vi "TREE_add symbol to tree.vi"(7 "symbol":i32, 10 "indentations to symbolize":i32, 11 "indentations in":i32[](array[numeric])) -> (3 "item symbols out":i32[](array[numeric]))   [LabVIEW 2014]
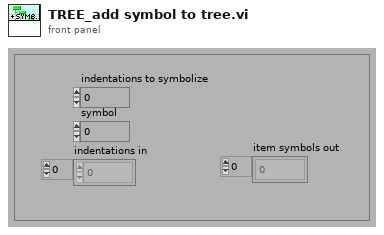
[diagram p1: front panel]
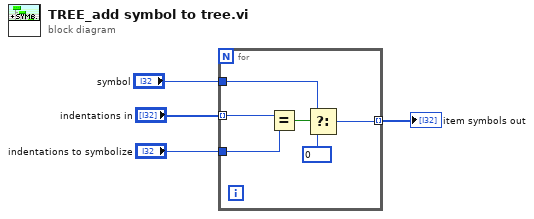
[diagram p0: block diagram]
diagram:
  n1 = for {
    tunnel: "indentations in" -> [w10] mode=indexing
    tunnel: "indentations to symbolize" -> [w8]
    tunnel: "symbol" -> [w7]
    tunnel: [w6] -> w1 mode=indexing
    n2 = Equal?(x=w10, y=w8) -> (x = y?=w9:bool)
    n3 = Select(t=w7, s=w9, f=0) -> (s? t:f=w6:i32)
  }
  "item symbols out" <- w1
